vi "example (graphs).vi"() -> ()   [LabVIEW 2021]
panel:
  out "Waveform Chart":dbl[][](graph)
  out "Waveform Graph":dbl[][](graph)
  in  "stop":bool
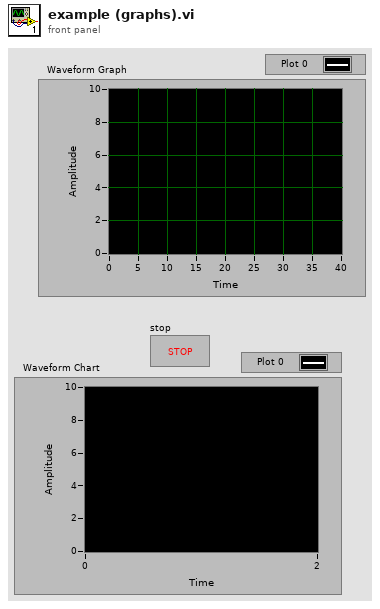
[diagram p1: front panel]
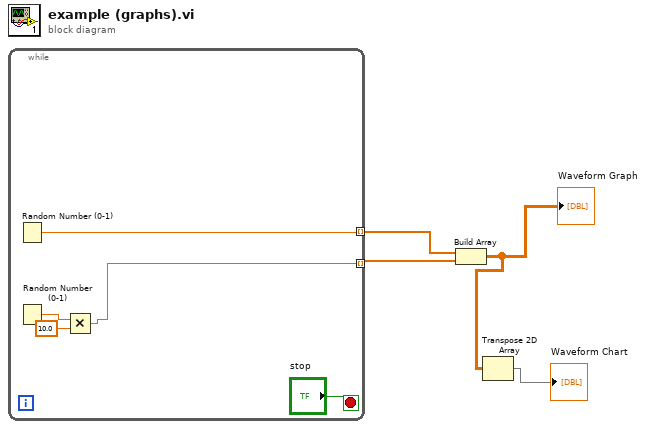
[diagram p0: block diagram]
diagram:
  n1 = while {
    tunnel: [w6] -> w3 mode=indexing
    tunnel: [w5] -> w4 mode=indexing
    stop <- "stop" stop-if-true
    n2 = Random Number (0-1)() -> (number: 0 to 1=w5:dbl)
    n3 = Random Number (0-1)() -> (number: 0 to 1=w8:dbl)
    n4 = Multiply(x=w8, y=10.0) -> (x*y=w6:dbl)
  }
  n5 = Build Array(w4, w3) -> (w2:dbl[][])
  "Waveform Graph" <- w2
  n6 = Transpose 2D Array(2D array=w2) -> (transposed array=→"Waveform Chart":dbl[][])
